vi "CLD 15 FGV for Text String Parsing Solution.vi"(8 "Error In":errorcluster, 11 "Mode":T2=enum."Read CSV") -> (0 "Error Out":errorcluster)   [LabVIEW 2009]
doc: "CLD 15 This challenge exercise creates an FGV from the CLD 15 solution. This VI reads the file and uses two sub-VI's to parse then format the file data for use."
uses:
  CLD 15 CSV file enum.ctl
  CLD 15 CSV file data structure.ctl
  <vilib>/Utility/file.llb/Read From Spreadsheet File (string).vi
  <vilib>/Utility/file.llb/Write To Spreadsheet File (string).vi
panel:
  out "Formatted Data Out":T1[](array[typedef])
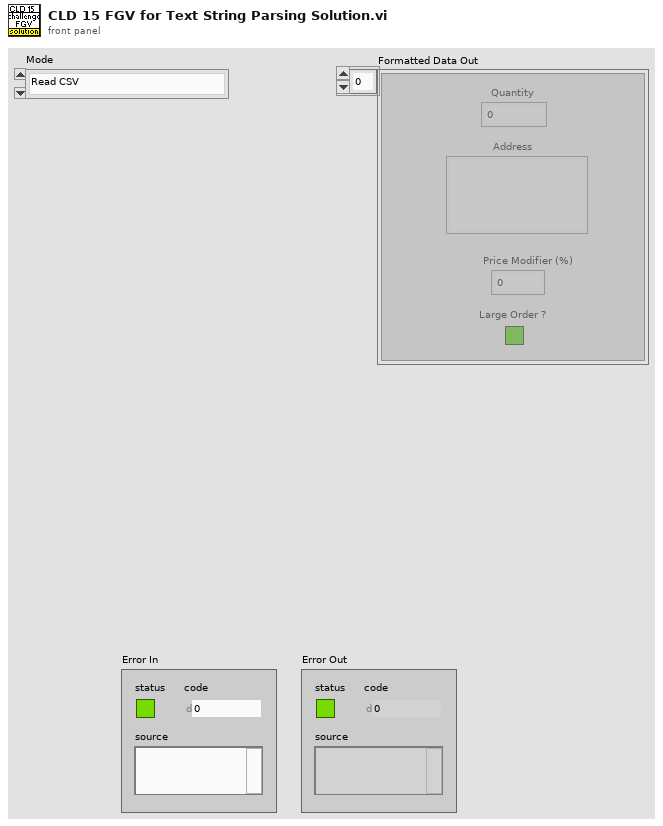
[diagram p1: front panel]
types:
  T1 = typedef "CLD 15 CSV file data structure.ctl" = cluster{"Quantity":i32, "Address":string, "Price Modifier (%)":dbl, "Large Order ?":bool}
  T2 = typedef "CLD 15 CSV file enum.ctl" = enum16{"initialize", "Read CSV", "Process Data", "Write CSV"}
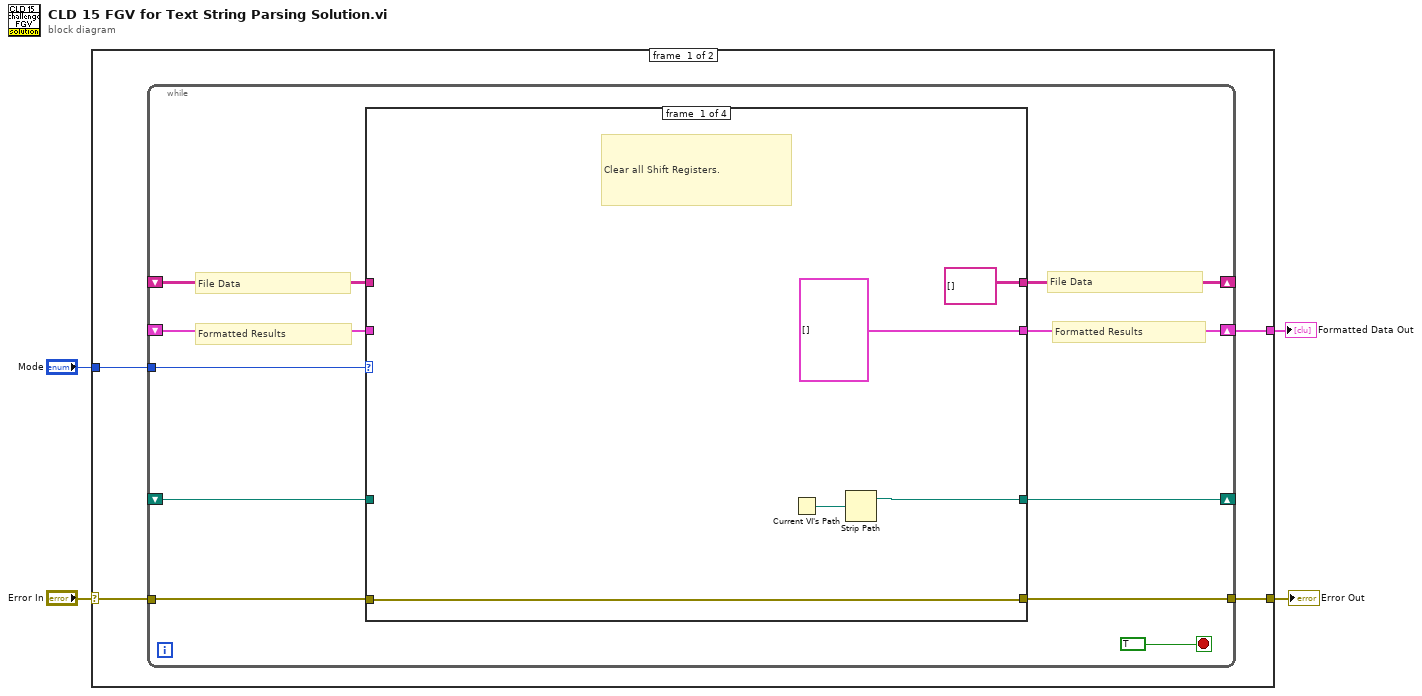
[diagram p0: block diagram]
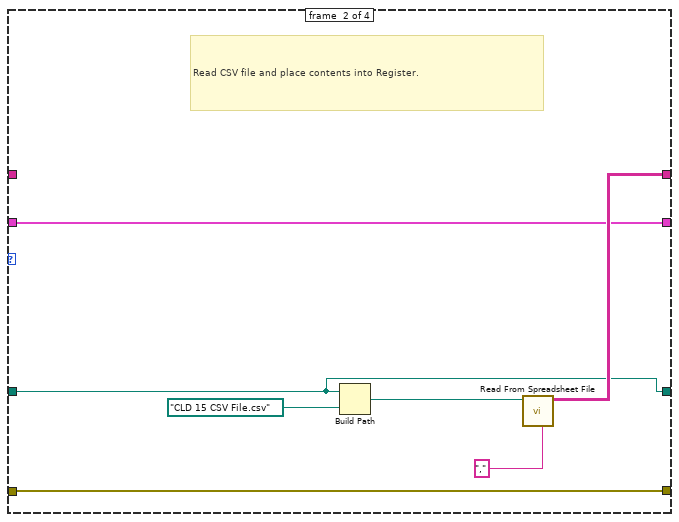
[diagram p2: hidden frame]
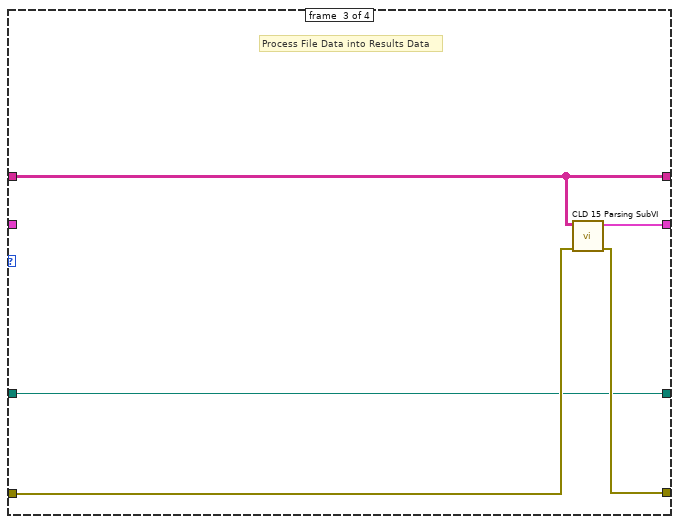
[diagram p3: hidden frame]
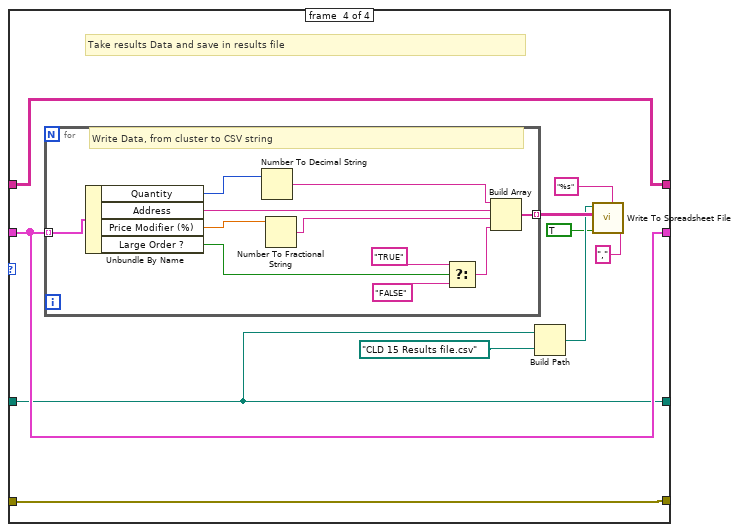
[diagram p4: hidden frame]
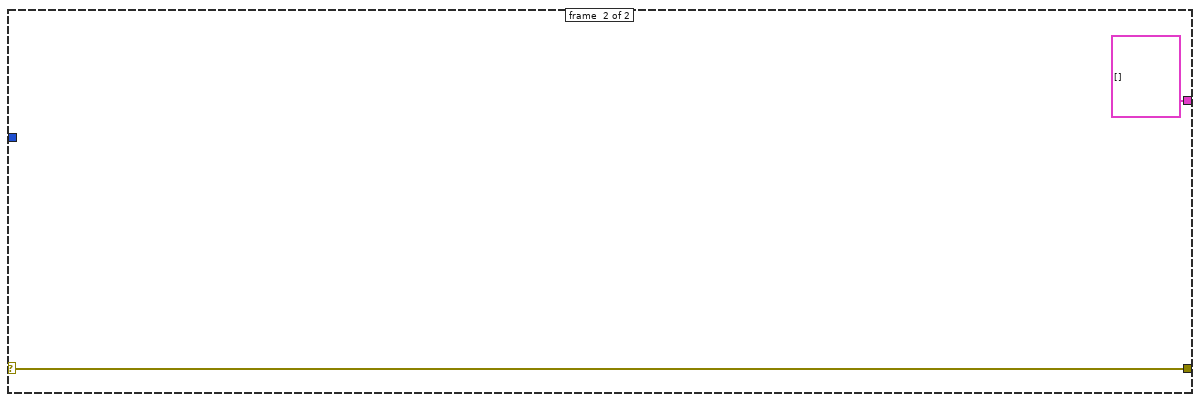
[diagram p5: hidden frame]
diagram:
  n1 = case shown="No Error" "Error In" {
    selector: "Error In" -> [w6 w58]
    tunnel: [w8 T1[] [] ("[Data In]")] -> w1
    tunnel: "Mode" -> [w7 _]
    tunnel: [w5 w58] -> w2
    frame #0 {
      n2 = while {
        tunnel: w7 -> [w17]
        tunnel: w6 -> [w16]
        tunnel: [w15] -> w5
        shift-right: [w18] -> w8
        shift-left: _ -> [w13]
        shift-right: [w12] -> _
        shift-left: _ -> [w11]
        shift-right: [w10] -> _
        shift-left: _ -> [w9]
        stop <- TRUE stop-if-true
        # "Formatted Results"
        # "File Data"
        # "Formatted Results"
        # "File Data"
        n3 = case shown="\"initialize\"" w17 {
          tunnel: w9 -> [_ w24 w31 w36]
          tunnel: [T1[] [] ("Data In") w27 w34 w38] -> w18
          tunnel: w16 -> [w21 w28 w33 w39]
          tunnel: [w21 w28 w32 w39] -> w15
          tunnel: w13 -> [_ w27 _ w38]
          tunnel: [string[][] [] ("all rows") w29 w35 w37] -> w12
          tunnel: w11 -> [_ _ w35 w37]
          tunnel: [w19 w24 w31 w36] -> w10
          frame #0 {
            # "Clear all Shift Registers."
            n4 = Current VI's Path() -> (path=w20:path)
            n5 = Strip Path(path=w20) -> (stripped path=w19:path)  [unwired: 1 out]
          }
          frame #1 {
            # "Read CSV file and place contents into Register."
            n6 = Build Path(base path=w24, name or relative path=path "CLD 15 CSV File.csv") -> (appended path=w25:path)
            n7 = call-poly <vilib>:"Read From Spreadsheet File.vi"("delimiter (\\t)"="," ("delimiter (\\t)"), "file path (dialog if empty)"=w25) -> ("all rows"=w29:string[][])  [unwired: 5 in, 4 out]
          }
          frame #2 {
            # "Process File Data into Results Data"
            n8 = call "CLD 15 Parsing SubVI.vi"("Error In"=w33, "all rows in"=w35) -> ("Error Out"=w32:errorcluster, "Data Out"=w34:T1[])  [unwired: 8 in]
          }
          frame #3 {
            # "Take results Data and save in results file"
            n9 = for {
              tunnel: [w47] -> w45 mode=indexing
              tunnel: w38 -> [w46] mode=indexing
              # "Write Data, from cluster to CSV string"
              n10 = Unbundle By Name(w46) -> ("Quantity"=w56:i32, "Address"=w50:string, "Price Modifier (%)"=w55:dbl, "Large Order ?"=w54:bool)
              n11 = Number To Decimal String(number=w56) -> (decimal integer string=w51:string)  [unwired: 1 in]
              n12 = Number To Fractional String(number=w55) -> (F-format string=w49:string)  [unwired: 3 in]
              n13 = Select(t="TRUE", s=w54, f="FALSE") -> (s? t:f=w48:string)
              n14 = Build Array(w51, w50, w49, w48) -> (w47:string[])
            }
            n15 = Build Path(base path=w36, name or relative path=path "CLD 15 Results file.csv") -> (appended path=w41:path)
            n16 = call-poly <vilib>:"Write To Spreadsheet File.vi"("delimiter (\\t)"="," ("delimiter (\\t)"), "format (%s)"="%s", "append to file? (new file:F)"=TRUE, "2D data"=w45, "file path (dialog if empty)"=w41) -> ()  [unwired: 3 in, 1 out]
          }
        }
      }
    }
    frame #1 {
    }
  }
  "Error Out" <- w2
  "Formatted Data Out" <- w1
